vi "sub_frame_to_packets.vi"(9 "packet size":i32=1600, 10 "Cluster":cluster{i32, "Data String":string}) -> (2 "packets":i16[][](array[numeric]))   [LabVIEW 2014]
panel:
  out "length":i32
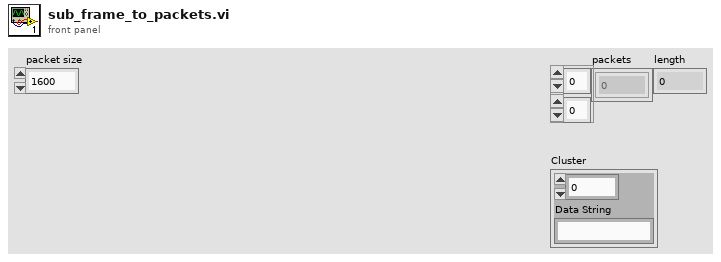
[diagram p1: front panel]
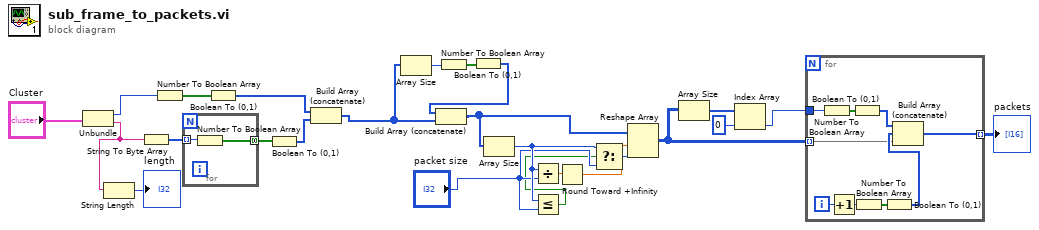
[diagram p0: block diagram]
diagram:
  n1 = Unbundle("Cluster") -> (w21:i32, "Data String"=w12:string)
  n2 = String Length(string=w12) -> (length=→"length":i32)
  n3 = String To Byte Array(string=w12) -> (unsigned byte array=w24:u8[])
  n4 = Number To Boolean Array(number=w21) -> (Boolean array=w22:bool[])
  n5 = for {
    tunnel: w24 -> [w27] mode=indexing
    tunnel: [w26] -> w23 mode=concatenating
    n6 = Number To Boolean Array(number=w27) -> (Boolean array=w26:bool[])
  }
  n7 = Boolean To (0,1)(Boolean=w22) -> (0, 1=w19:i16[])
  n8 = Boolean To (0,1)(Boolean=w23) -> (0, 1=w20:i16[])
  n9 = Build Array (concatenate)(w19, w20) -> (w1:i16[])
  n10 = Array Size(array=w1) -> (size(s)=w5:i32)
  n11 = Number To Boolean Array(number=w5) -> (Boolean array=w4:bool[])
  n12 = Boolean To (0,1)(Boolean=w4) -> (0, 1=w2:i16[])
  n13 = Build Array (concatenate)(w2, w1) -> (w3:i16[])
  n14 = Array Size(array=w3) -> (size(s)=w8:i32)
  n15 = Divide(x=w8, y="packet size") -> (x/y=w18:dbl)
  n16 = Less Or Equal?(x=w8, y="packet size") -> (x <= y?=w6:bool)
  n17 = Round Toward +Infinity(x=w18) -> (ceil(x): smallest int >= x=w10:dbl)
  n18 = Select(t=w8, s=w6, f="packet size") -> (s? t:f=w9:i32)
  n19 = Reshape Array(w3, w10, w9) -> (w17:i16[][])
  n20 = Array Size(array=w17) -> (size(s)=w15:i32[])
  n21 = Index Array(array=w15, index=0) -> (element=w14:i32)
  n22 = for {
    tunnel: w17 -> [w33] mode=indexing
    tunnel: w14 -> [w31]
    tunnel: [w28] -> w16 mode=indexing
    i -> [w35]
    n23 = Number To Boolean Array(number=w31) -> (Boolean array=w32:bool[])
    n24 = Increment(x=w35) -> (x+1=w29:i32)
    n25 = Boolean To (0,1)(Boolean=w32) -> (0, 1=w30:i16[])
    n26 = Number To Boolean Array(number=w29) -> (Boolean array=w36:bool[])
    n27 = Boolean To (0,1)(Boolean=w36) -> (0, 1=w34:i16[])
    n28 = Build Array (concatenate)(w30, w34, w33) -> (w28:i16[])
  }
  "packets" <- w16
